vi "absolute_timing_sequence_to_waveform_data.vi"(0 "Variable Names":string[](array[string]), 1 "Clock Rate":dbl, 3 "Timing Sequence Control (ms)":string[][](array[string]), 5 "Current Value Array":dbl[](array[numeric]), 11 "Force waveform length to be multiple of 2\n(Necessary on old hardware)":bool, 14 "units/sec (ms=1000)":dbl) -> (4 "Transitions":u32[](array[numeric]), 6 "Data":u32[](array[numeric]) format="%04b", 8 "Waveform was padded":bool, 10 "output waveform":digitaldata, 15 "Waveform Duration (ms)":dbl)   [LabVIEW 2013]
uses:
  <vilib>/gmath/NI_Gmath.lvlib
panel:
  out "Gap Timing Sequence [ms]":dbl[][](array[numeric])
  out "Absolute Timing Sequence [samples]":dbl[][](array[numeric])
  out "Flattened Transition Array":u64[](array[numeric])
  out "Redunancy Removed":u64[](array[numeric])
  out "Non-Redundant Sorted Array":u64[](array[numeric])
  out "Last Element Reduced":u32[](array[numeric])
  out "# of Channels":i32
  out "# transitions per channel":i32
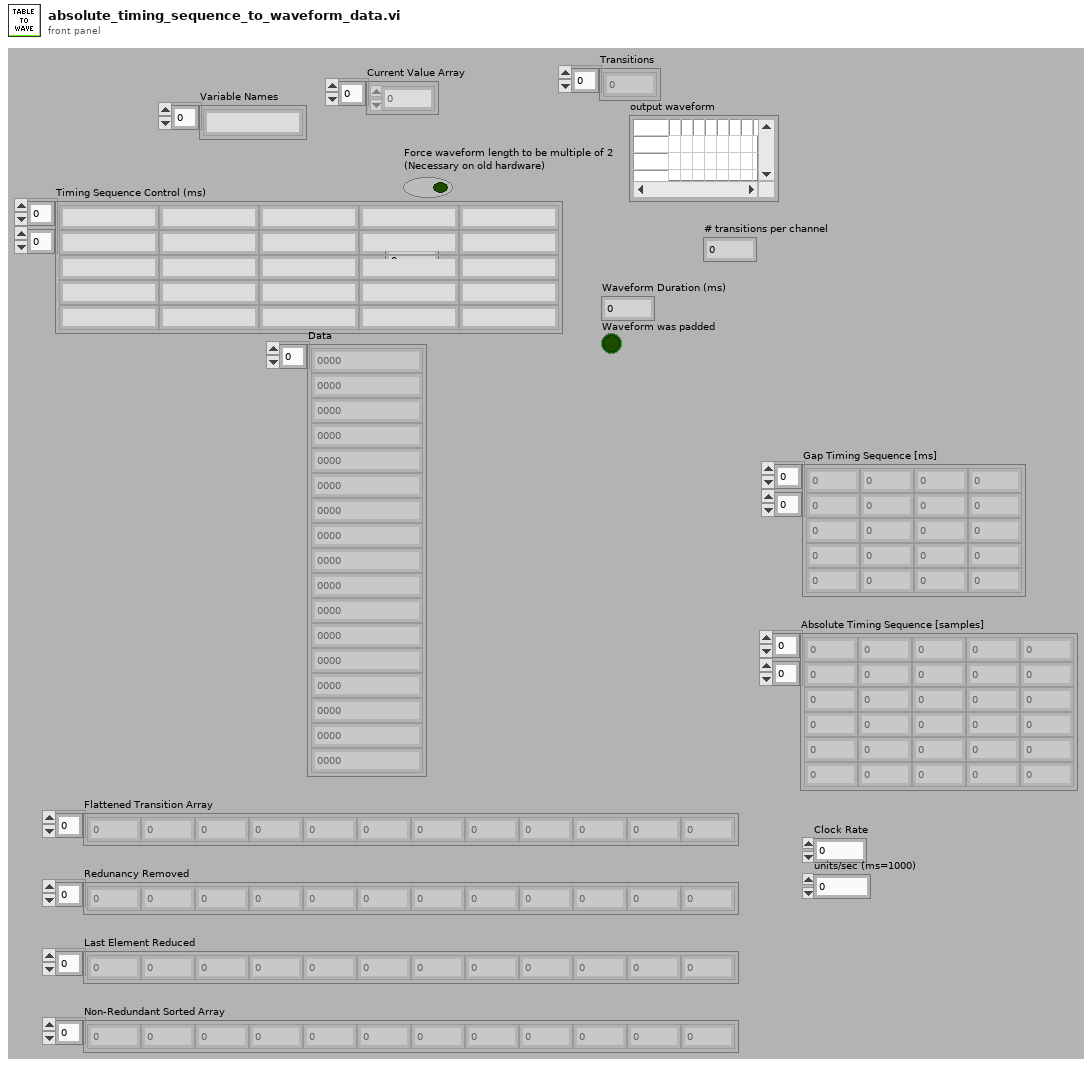
[diagram p1: front panel]
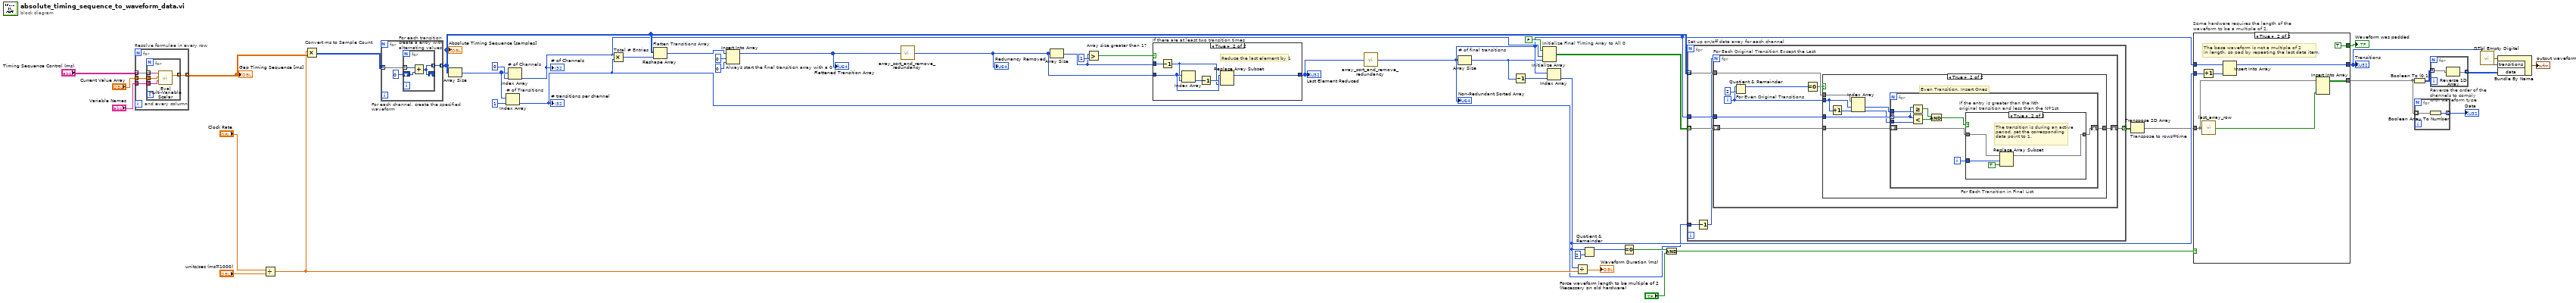
[diagram p0: block diagram]
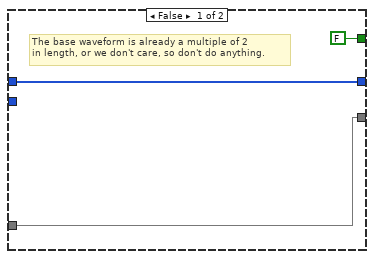
[diagram p2: hidden frame]
diagram:
  n1 = for "Resolve formulae in every row" {
    tunnel: "Timing Sequence Control (ms)" -> [w50] mode=indexing
    tunnel: [w47] -> w45 mode=indexing
    tunnel: "Variable Names" -> [w49]
    tunnel: "Current Value Array" -> [w48]
    n2 = for "and every column" {
      tunnel: w50 -> [w54] mode=indexing
      tunnel: [w52] -> w47 mode=indexing
      tunnel: w49 -> [w53]
      tunnel: w48 -> [w51]
      n3 = call <vilib>:"Eval Multi-Variable Scalar.vi"("Variables"=w53, "X Values"=w51, "formula"=w54) -> ("y value"=w52:dbl)  [unwired: 1 in, 1 out]
    }
  }
  "Gap Timing Sequence [ms]" <- w45
  n4 = Divide(x="Clock Rate", y="units/sec (ms=1000)") -> (x/y=w26:dbl)
  n5 = Multiply "Convert ms to Sample Count"(x=w26, y=w45) -> (x*y=w46:u32[][])
  n6 = for "For each channel, create the specified waveform" {
    tunnel: w46 -> [w57] mode=indexing
    tunnel: [w55] -> w32 mode=indexing
    n7 = for "For each transition create a entry with alternating values" {
      tunnel: w57 -> [w60] mode=indexing
      shift-right: [w58] -> _
      shift-left: u64 0 -> [w59]
      tunnel: [w58] -> w55 mode=indexing
      n8 = Add(x=w60, y=w59) -> (x+y=w58:u64)
    }
  }
  "Absolute Timing Sequence [samples]" <- w32
  n9 = Array Size(array=w32) -> (size(s)=w44:i32[])
  n10 = Index Array "# of Transitions"(array=w44, index=1) -> (element=w1:i32)
  "# transitions per channel" <- w1
  n11 = Index Array "# of Channels"(array=w44, index=0) -> (element=w2:i32)
  "# of Channels" <- w2
  n12 = Multiply "Total # Entries"(x=w2, y=w1) -> (x*y=w41:i32)
  n13 = Reshape Array "Flatten Transitions Array"(w32, w41) -> (w39:u64[])
  n14 = Insert Into Array "Always start the final transition array with a 0"(array=w39, index=u32 0, new element=u64 0 ("new element/subarray")) -> (w36:u64[])
  "Flattened Transition Array" <- w36
  n15 = call "array_sort_and_remove_redundancy.vi"("Full Array"=w36) -> ("Non-Redundant Sorted Array"=w24:u32[])
  "Redunancy Removed" <- w24
  n16 = Array Size(array=w24) -> (size(s)=w23:i32)
  n17 = Greater? "Array size greater than 1?"(x=w23, y=1) -> (0:w22:bool)
  n18 = case "If there are at least two transition times" shown="True" w22 {
    tunnel: w24 -> [w61 w66]
    tunnel: w23 -> [_ w67]
    tunnel: [w61 w62] -> w35
    frame False {
      # "The only element is zero, just leave it."
    }
    frame True {
      # "Reduce the last element by 1"
      n19 = Decrement(x=w67) -> (x-1=w65:i32)
      n20 = Index Array(array=w66, index=w65) -> (element=w64:u32)
      n21 = Decrement(x=w64) -> (x-1=w63:u32)
      n22 = Replace Array Subset "Replace Array Subset"(array=w66, new element=w63, index=w65) -> (w62:u32[])
    }
  }
  "Last Element Reduced" <- w35
  n23 = call "array_sort_and_remove_redundancy.vi"("Full Array"=w35) -> ("Non-Redundant Sorted Array"=w15:u32[])
  "Non-Redundant Sorted Array" <- w15
  n24 = Array Size "# of final transitions"(array=w15) -> (size(s)=w12:i32)
  n25 = Decrement(x=w12) -> (x-1=w27:i32)
  n26 = Initialize Array "Initialize Final Timing Array to All 0"(FALSE, w2, w12) -> (w33:bool[][])
  n27 = Index Array(array=w15, index=w27) -> (element=w16:u32)
  n28 = Divide(x=w16, y=w26) -> (x/y=→"Waveform Duration (ms)":dbl)
  n29 = Quotient & Remainder(x=w16, y=u32 2) -> (x-y*floor(x/y)=w21:u32)  [unwired: 1 out]
  n30 = Equal To 0?(x=w21) -> (x = 0?=w19:bool)
  n31 = And(x=w19, y="Force waveform length to be multiple of 2\n(Necessary on old hardware)") -> (x .and. y?=w17:bool)
  n32 = for "Set up on/off data array for each channel" {
    tunnel: w33 -> [w73] mode=indexing
    tunnel: w32 -> [w72] mode=indexing
    tunnel: [w71] -> w11 mode=indexing
    tunnel: w15 -> [w70]
    tunnel: w1 -> [w68]
    n33 = Decrement(x=w68) -> (x-1=w69:i32)
    n34 = for "For Each Original Transition Except the Last" {
      N: w69 -> [_]
      tunnel: w72 -> [w79]
      tunnel: w70 -> [w74]
      shift-right: [w78] -> w71
      shift-left: w73 -> [w80]
      i -> [w75]
      n35 = Quotient & Remainder "For Even Original Transitions"(x=w75, y=2) -> (x-y*floor(x/y)=w77:i32)  [unwired: 1 out]
      n36 = Equal To 0?(x=w77) -> (x = 0?=w76:bool)
      n37 = case shown="True" w76 {
        tunnel: w80 -> [w82 w90]
        tunnel: w79 -> [_ w87]
        tunnel: [w82 w89] -> w78
        tunnel: w75 -> [_ w88]
        tunnel: w74 -> [_ w85]
        frame False {
          # "Odd Transition, Do Nothing"
        }
        frame True {
          # "Even Transition, Insert Ones"
          n38 = Increment(x=w88) -> (x+1=w84:i32)
          n39 = Index Array "Index Array"(array=w87, index #1=w88, index #2=w84) -> (element #1=w86:u64, element #2=w83:u64)
          n40 = for "For Each Transition in Final List" {
            tunnel: w83 -> [w98]
            tunnel: w86 -> [w97]
            tunnel: w85 -> [w96] mode=indexing
            shift-right: [w99] -> w89
            shift-left: w90 -> [w92]
            i -> [w91]
            n41 = Greater Or Equal?(x=w96, y=w97) -> (x >= y?=w95:bool)
            n42 = Less?(x=w96, y=w98) -> (x < y?=w94:bool)
            n43 = And(x=w95, y=w94) -> (x .and. y?=w93:bool)
            n44 = case "If the entry is greater than the Nth\noriginal transition and less than the N+1st" shown="True" w93 {
              tunnel: w92 -> [w100 w104]
              tunnel: [w100 w103] -> w99
              tunnel: w91 -> [_ w102]
              frame False {
                # "Do nothing."
              }
              frame True {
                # "The transition is during an active period, set the corresponding data point to 1."
                n45 = Replace Array Subset(array=w104, new element=TRUE, index=w102) -> (w103:bool[])
              }
            }
          }
        }
      }
    }
  }
  n46 = Transpose 2D Array "Transpose to rows=time"(2D array=w11) -> (transposed array=w9:bool[][])
  n47 = case "Some hardware requires the length of the\nwaveform to be a multiple of 2." shown="True" w17 {
    tunnel: w16 -> [_ w115]
    tunnel: w15 -> [w107 w113]
    tunnel: [w107 w112] -> w7
    tunnel: w9 -> [w106 w110]
    tunnel: [w106 w109] -> w8
    tunnel: [FALSE TRUE] -> w14
    frame False {
      # "The base waveform is already a multiple of 2\nin length, or we don't care, so don't do anything."
    }
    frame True {
      # "The base waveform is not a multiple of 2\nin length, so pad by repeating the last data item."
      n48 = Increment(x=w115) -> (x+1=w114:u32)
      n49 = call "last_array_row.vi"("array"=w110) -> ("subarray"=w111:bool[])
      n50 = Insert Into Array(array=w113, new element=w114) -> (w112:u32[])  [unwired: 1 in]
      n51 = Insert Into Array(array=w110, new element=w111) -> (w109:bool[][])  [unwired: 2 in]
    }
  }
  "Waveform was padded" <- w14
  "Transitions" <- w7
  n52 = Boolean To (0,1)(Boolean=w8) -> (0, 1=w5:i16[][])
  n53 = for {
    tunnel: w8 -> [w117] mode=indexing
    tunnel: [w116] -> w10 mode=indexing
    n54 = Boolean Array To Number(Boolean array=w117) -> (number=w116:u32)
  }
  "Data" <- w10
  n55 = for "Reverse the order of the \nchannels to comply \nwith waveform type" {
    tunnel: w5 -> [w119] mode=indexing
    tunnel: [w118] -> w4 mode=indexing
    n56 = Reverse 1D Array(array=w119) -> (reversed array=w118:i16[])
  }
  n57 = call <vilib>:"DTbl Empty Digital.vi"() -> ("digital data"=w6:digitaldata)  [unwired: 5 in]
  n58 = Bundle By Name(cluster=w6, "transitions"=w7, "data"=w4) -> (→"output waveform":digitaldata)
